vi "decodeStream.vi"(8 "error in (no error)":errorcluster, 9 "beginIndex":i32, 10 "binary stream":u8[](array[numeric]), 11 "tBSONBoolean in":refnum<class "tBSONBoolean.lvclass">) -> (0 "error out":errorcluster, 1 "endIndex":i32, 2 "binary stream out":u8[](array[numeric]), 3 "tBSONBoolean out":refnum<class "tBSONBoolean.lvclass">)   [LabVIEW 2013, in "BSON.lvlib" / "tBSONBoolean.lvclass"]
uses:
  tBSONBoolean.lvclass
  tBSONElement/tBSONElement.lvclass
  status.ctl
  setValue.vi
  BSON.lvlib
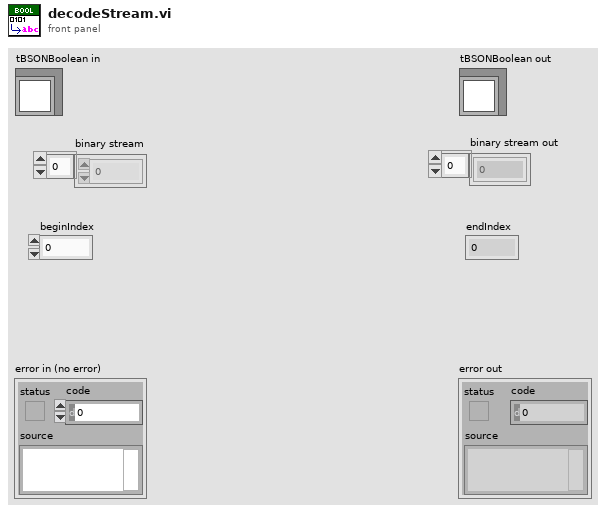
[diagram p1: front panel]
types:
  T1 = typedef "BSON.lvlib/status.ctl" = enum16{"Stream Corrupted or Ended Abruptly", "Incorrect Type In Stream", "ObjectID Invalid", "Method Not Implemented", "Invalid Name", "Invalid URI", "AutoReconnect", "Operation Failed", "Incorrectly Configured", "Cursor Not Found", "Timeout", "Invalid Type", "Empty Name", "Duplicate Name", "MD5Incorrect"}
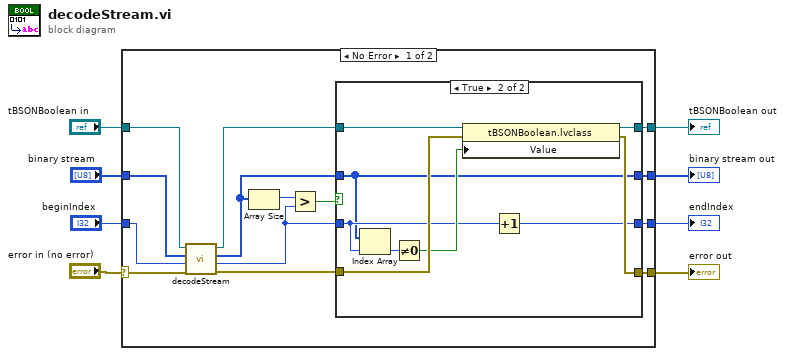
[diagram p0: block diagram]
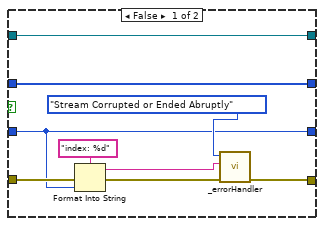
[diagram p2: hidden frame]
diagram:
  n1 = case shown="No Error" "error in (no error)" {
    selector: "error in (no error)" -> [w22 w44]
    tunnel: [w18 w44] -> w4
    tunnel: "beginIndex" -> [w20 w43]
    tunnel: [w15 w43] -> w3
    tunnel: "binary stream" -> [w13 w42]
    tunnel: [w12 w42] -> w2
    tunnel: "tBSONBoolean in" -> [w21 w41]
    tunnel: [w17 w41] -> w1
    frame No Error {
      n2 = call-parent "decodeStream.vi"("error in (no error)"=w22, "beginIndex"=w20, "binary stream"=w13, "tBSONElement in"=w21) -> ("error out"=w16:errorcluster, "endIndex"=w11:i32, "binary stream out"=w9:u8[], "tBSONElement out"=w19:refnum<class "tBSONBoolean.lvclass">)  [unwired: 4 in]
      n3 = Array Size(array=w9) -> (size(s)=w14:i32)
      n4 = Greater?(x=w14, y=w11) -> (0:w10:bool)
      n5 = case shown="True" w10 {
        tunnel: w19 -> [w31 w40]
        tunnel: [w23 w39] -> w18
        tunnel: [w31 w38] -> w17
        tunnel: w16 -> [w29 w37]
        tunnel: [w24 w34] -> w15
        tunnel: w11 -> [w24 w33]
        tunnel: w9 -> [w30 w32]
        tunnel: [w30 w32] -> w12
        frame False {
          n6 = Format Into String(format string="index: %d", error in=w29, w24) -> (resulting string=w26:string, error out=w27:errorcluster)  [unwired: 1 in]
          n7 = call "_errorHandler.vi"("error in (no error)"=w27, "Additional Text"=w26, "Error Type"=status."Stream Corrupted or Ended Abruptly") -> ("error out"=w23:errorcluster)  [unwired: 8 in]
        }
        frame True {
          n8 = Index Array(array=w32, index=w33) -> (element=w36:u8)
          n9 = Not Equal To 0?(x=w36) -> (x != 0?=w35:bool)
          n10 = property class="tBSONBoolean.lvclass"(reference=w40, error in=w37, "Value"=w35) -> (reference out=w38:refnum<class "tBSONBoolean.lvclass">, error out=w39:errorcluster)
          n11 = Increment(x=w33) -> (x+1=w34:i32)
        }
      }
    }
    frame Error {
    }
  }
  "error out" <- w4
  "tBSONBoolean out" <- w1
  "binary stream out" <- w2
  "endIndex" <- w3
